vi "Kinect Extract Mouse 2.vi"(0 "Image Src":T1, 1 "Image Mask":T1, 2 "Cropped Image Src":T1, 3 "Particle Report":T2, 5 "error in (no error)":errorcluster, 7 "Width":i32=100, 9 "Height":i32=100) -> (14 "Extracted Particle":T1, 19 "error out":errorcluster)   [LabVIEW 2011]
uses:
  <vilib>/vision/Image Controls.llb/IMAQ Image.ctl
  <vilib>/vision/NI_Vision_Development_Module.lvlib
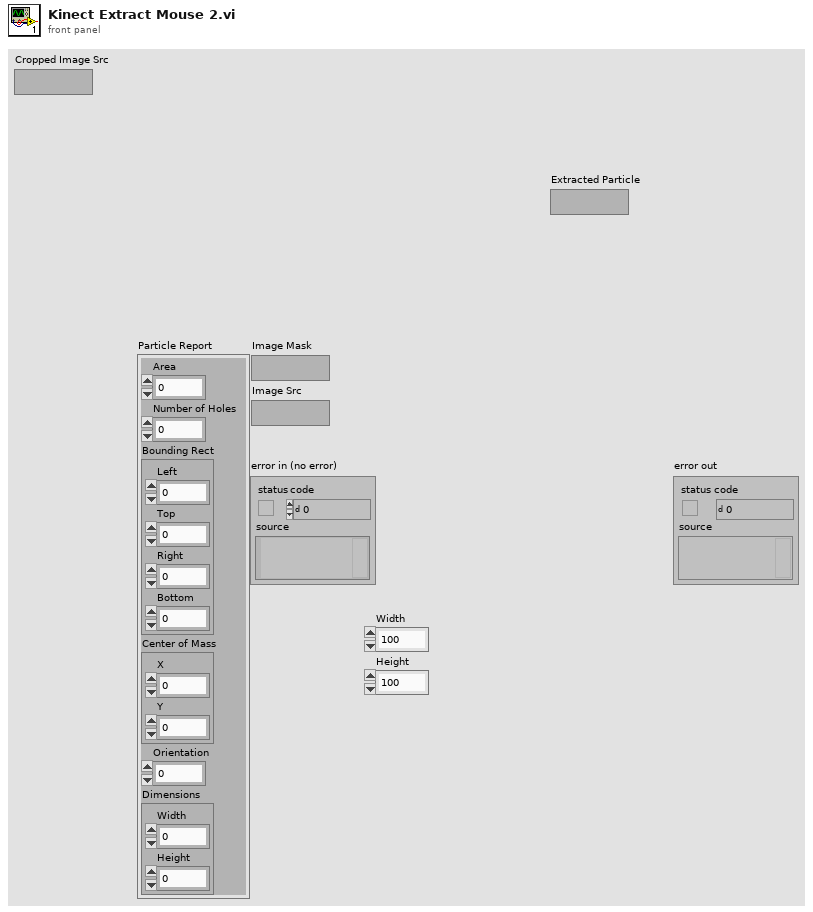
[diagram p1: front panel]
types:
  T1 = typedef "IMAQ Image.ctl" = refnum<image>
  T2 = cluster{"Area":dbl, "Number of Holes":dbl, "Bounding Rect":cluster{"Left":dbl, "Top":dbl, "Right":dbl, "Bottom":dbl}, "Center of Mass":cluster{"X":dbl, "Y":dbl}, "Orientation":dbl, "Dimensions":cluster{"Width":dbl, "Height":dbl}}
  T3 = typedef "Image Type" = u32
  T4 = cluster{"Left":dbl, "Top":dbl, "Right":dbl, "Bottom":dbl}
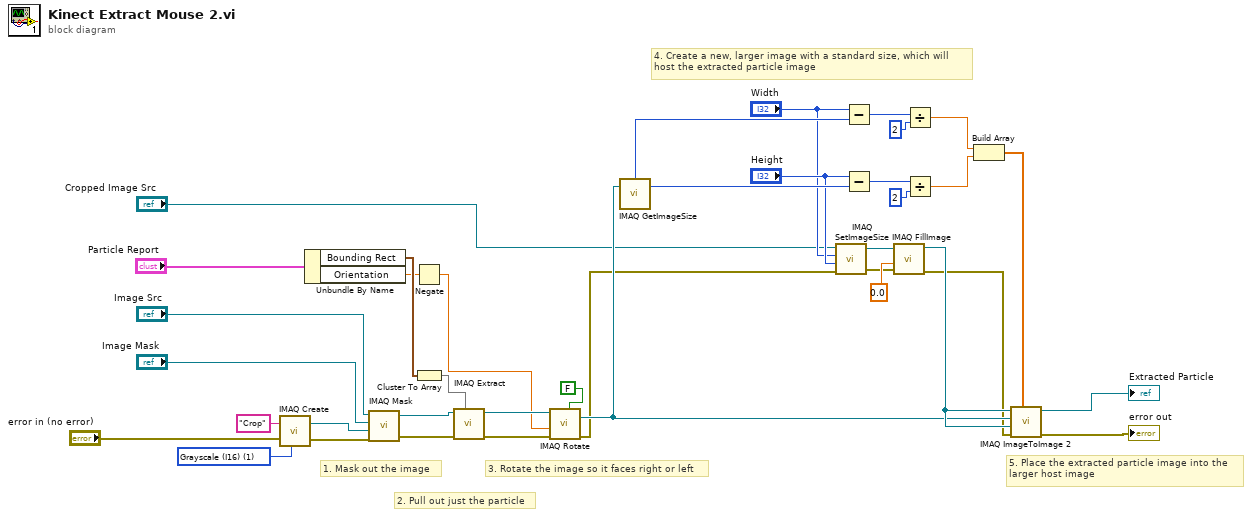
[diagram p0: block diagram]
diagram:
  w6 = T3 1 items=["Grayscale (U8)", "Grayscale (I16)", "Grayscale (SGL)", "Complex (CSG)", "RGB (U32)", "HSL (U32)", "RGB (U64)", "Grayscale (U16)"] ("Image Type")
  # "5. Place the extracted particle image into the\nlarger host image"
  # "4. Create a new, larger image with a standard size, which will\nhost the extracted particle image"
  # "3. Rotate the image so it faces right or left"
  # "2. Pull out just the particle"
  # "1. Mask out the image"
  n1 = call "IMAQ Create"("Image Name"="Crop", "Image Type"=w6, "error in (no error)"="error in (no error)") -> ("New Image"=w3:T1, "error out"=w4:errorcluster)  [unwired: 2 in]
  n2 = Unbundle By Name("Particle Report") -> ("Bounding Rect"=w37:T4, "Orientation"=w33:dbl)
  n3 = call "IMAQ Mask"("error in (no error)"=w4, "Image Dst"=w3, "Image Mask"="Image Mask", "Image Src"="Image Src") -> ("error out"=w28:errorcluster, "Image Dst Out"=w38:T1)  [unwired: 1 in]
  n4 = Negate(x=w33) -> (-x=w32:dbl)
  n5 = Cluster To Array(cluster=w37) -> (array=w36:dbl[])
  n6 = call "IMAQ Extract"("Optional Rectangle"=w36, "error in (no error)"=w28, "Image Src"=w38) -> ("error out"=w27:errorcluster, "Image Dst Out"=w35:T1)  [unwired: 7 in]
  n7 = call "IMAQ Rotate"("Maintain Size"=FALSE, "error in (no error)"=w27, "Angle (degrees)"=w32, "Image Src"=w35) -> ("error out"=w2:errorcluster, "Image Dst Out"=w11:T1)  [unwired: 6 in]
  n8 = call "IMAQ GetImageSize"("Image"=w11) -> ("Y Resolution"=w18:i32, "X Resolution"=w19:i32)  [unwired: 3 in, 1 out]
  n9 = call "IMAQ SetImageSize"("error in (no error)"=w2, "Y Resolution"="Height", "X Resolution"="Width", "Image"="Cropped Image Src") -> ("error out"=w15:errorcluster, "Image Out"=w17:T1)  [unwired: 1 in]
  n10 = Subtract(x="Width", y=w19) -> (x-y=w23:i32)
  n11 = Subtract(x="Height", y=w18) -> (x-y=w24:i32)
  n12 = call "IMAQ FillImage"("error in (no error)"=w15, "Pixel Value (U8, U16, I16, Float)"=sgl 0.0, "Image"=w17) -> ("error out"=w10:errorcluster, "Image Out"=w14:T1)  [unwired: 7 in]
  n13 = Divide(x=w23, y=2) -> (x/y=w22:dbl)
  n14 = Divide(x=w24, y=2) -> (x/y=w21:dbl)
  n15 = Build Array(w22, w21) -> (w20:dbl[])
  n16 = call "IMAQ ImageToImage 2"("Offset Left/Top"=w20, "error in (no error)"=w10, "Image Dst"=w14, "Image Src (Small)"=w11, "Image Src (Large)"=w14) -> ("error out"=→"error out":errorcluster, "Image Dst Out"=→"Extracted Particle":T1)  [unwired: 5 in]
